vi "Model 3566-Wait For Read.vi"(8 "error in":errorcluster, 11 "Wait For Read(ms)":u32) -> (0 "error out":errorcluster)   [LabVIEW 2018]
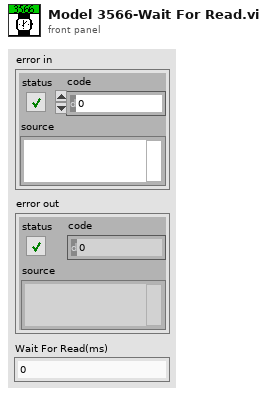
[diagram p1: front panel]
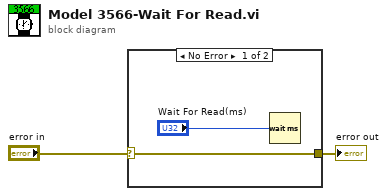
[diagram p0: block diagram]
diagram:
  n1 = case shown="No Error" "error in" {
    selector: "error in" -> [w4 w5]
    tunnel: [w4 w5] -> w2
    frame No Error {
      n2 = Wait (ms)(milliseconds to wait="Wait For Read(ms)") -> ()  [unwired: 1 out]
    }
    frame Error {
    }
  }
  "error out" <- w2
